vi "Write Settings.vi"(8 "error in (no error)":errorcluster, 10 "Settings":T5, 11 "Tool Data in":refnum<class "Tool Data.lvclass">) -> (0 "error out":errorcluster, 3 "Tool Data out":refnum<class "Tool Data.lvclass">)   [LabVIEW 2019, in "Tool Data.lvclass"]
uses:
  Tool Data.lvclass
  Settings/Dot Settings/Dot Settings.lvclass
  Settings/Setting Database/Typedefs/PublicEvents--Setting Database.DotsUpdated.ctl
  Settings/Setting Database/Setting Database.lvclass
  Settings/Funnel Settings/Funnel Settings.lvclass
  Settings/Setting Database/Typedefs/PublicEvents--Setting Database.FunnelsUpdated.ctl
  Settings/Rectangle Settings/Rectangle Settings.lvclass
  Settings/Setting Database/Typedefs/PublicEvents--Setting Database.RectanglesUpdated.ctl
  Settings/Path Settings/Path Settings.lvclass
  Settings/Setting Database/Typedefs/PublicEvents--Setting Database.PathsUpdated.ctl
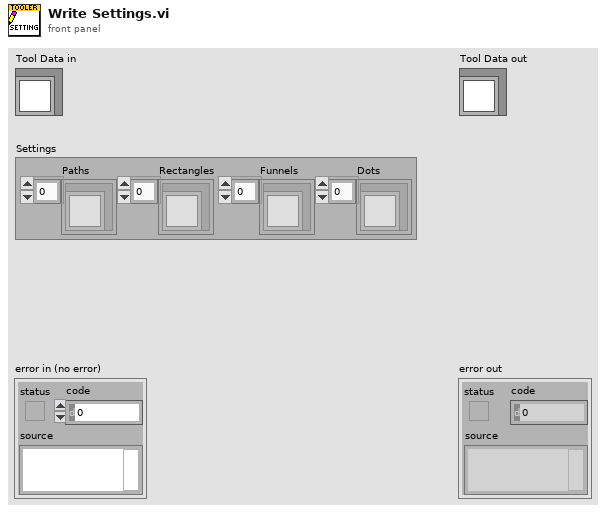
[diagram p1: front panel]
types:
  T1 = typedef "Setting Database.lvclass/PublicEvents--Setting Database.PathsUpdated.ctl" = refnum<class "Path Settings.lvclass">[]
  T2 = typedef "Setting Database.lvclass/PublicEvents--Setting Database.RectanglesUpdated.ctl" = refnum<class "Rectangle Settings.lvclass">[]
  T3 = typedef "Setting Database.lvclass/PublicEvents--Setting Database.FunnelsUpdated.ctl" = refnum<class "Funnel Settings.lvclass">[]
  T4 = typedef "Setting Database.lvclass/PublicEvents--Setting Database.DotsUpdated.ctl" = refnum<class "Dot Settings.lvclass">[]
  T5 = cluster{"Paths":T1, "Rectangles":T2, "Funnels":T3, "Dots":T4}
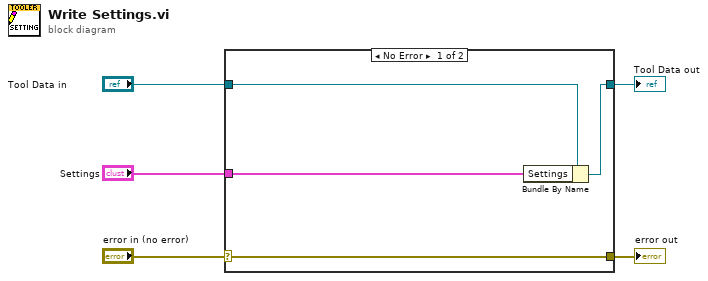
[diagram p0: block diagram]
diagram:
  n1 = case shown="No Error" "error in (no error)" {
    selector: "error in (no error)" -> [w9 w10]
    tunnel: [w9 w10] -> w4
    tunnel: [w7 w11] -> w2
    tunnel: "Tool Data in" -> [w8 w11]
    tunnel: "Settings" -> [w6 _]
    frame No Error {
      n2 = Bundle By Name(cluster=w8, "Settings"=w6) -> (w7:refnum<class "Tool Data.lvclass">)
    }
    frame Error {
    }
  }
  "error out" <- w4
  "Tool Data out" <- w2
